vi "Day 1.vi"() -> ()   [LabVIEW 2023]
panel:
  out "top 3":i32
  out "MAX":i32
  in  "Input":string="22243\n11899\n\n1696\n2595\n5331\n6092\n5274\n5641\n1345\n6626\n2005\n6260\n6410\n2092\n3501\n\n3982\n4505\n5836\n6059\n6513\n1151\n\n7002\n6597\n7174\n3618\n4734\n5107\n1388\n6493\n6541\n6440\n5291\n4492\n\n1341\n6520\n8531\n3483\n9221\n2847\n3930\n4012\n\n4074\n2101\n2200\n1333\n2991\n3186\n6711\n2248\n6655\n\n5102\n2672\n2842\n2274\n6828\n3765\n5290\n6004\n7237\n1509\n3128\n1593\n\n8404\n7548\n4075\n8246\n5590\n2107\n1204\n6374\n1865\n5657\n\n62852\n\n10643\n5981\n9631\n1574\n2962\n1021\n9811\n1566\n\n2027\n1193\n1487\n4493\n6215\n3315\n1353\n3703\n3987\n8158\n\n5969\n3824\n4696\n6948\n5098\n1364\n5943\n2489\n3523\n2585\n3242\n5724\n\n2113\n1381\n4067\n2344\n4778\n2645\n3968\n6599\n6451\n4462\n3882\n2312\n3843\n\n294..."
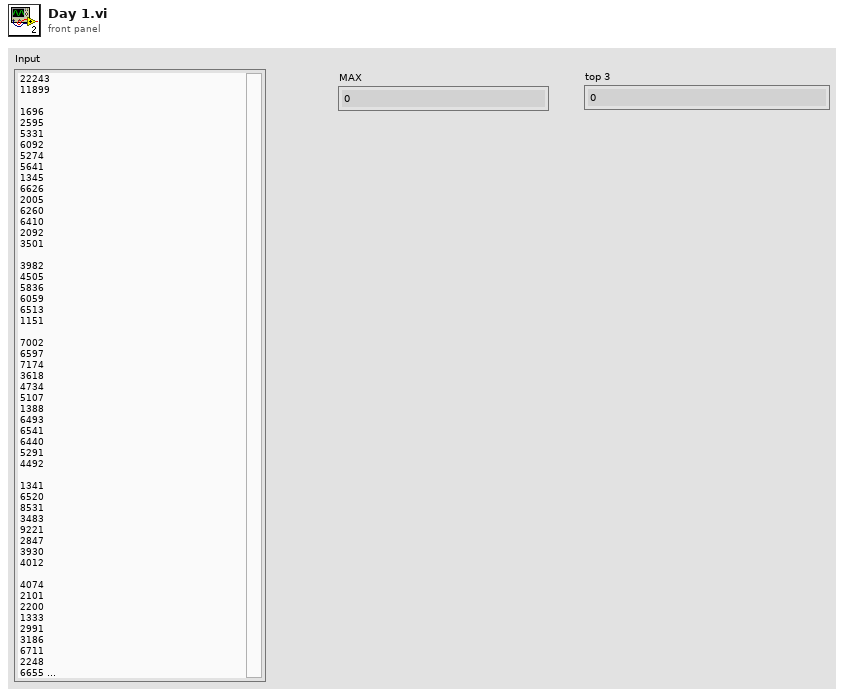
[diagram p1: front panel]
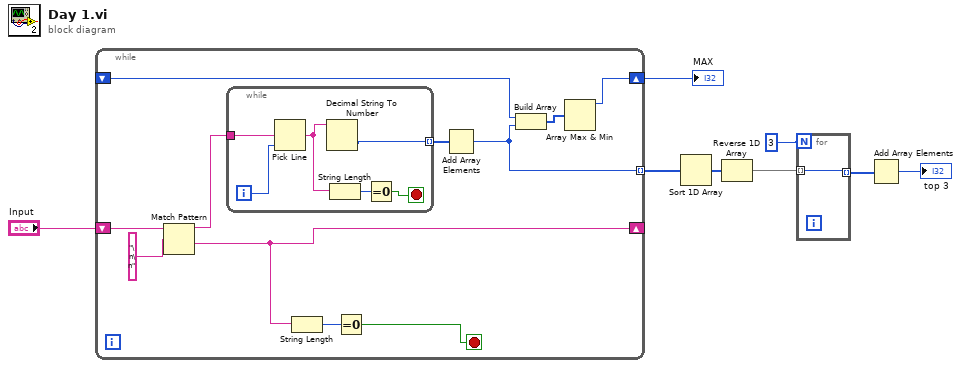
[diagram p0: block diagram]
diagram:
  n1 = while {
    shift-right: [w16] -> _
    shift-left: "Input" -> [w19]
    shift-right: [w11] -> w7
    shift-left: _ -> [w10]
    tunnel: [w9] -> w6 mode=indexing
    stop <- w15 stop-if-true
    n2 = Match Pattern(string=w19, regular expression="\n\n") -> (before substring=w14:string, after substring=w16:string)  [unwired: 1 in, 2 out]
    n3 = while {
      tunnel: w14 -> [w23]
      tunnel: [w24] -> w13 mode=indexing
      i -> [w25]
      stop <- w21 stop-if-true
      n4 = Pick Line(multi-line string=w23, line index=w25) -> (output string=w20:string)  [unwired: 1 in]
      n5 = Decimal String To Number(string=w20) -> (number=w24:i32)  [unwired: 2 in, 1 out]
      n6 = String Length(string=w20) -> (length=w22:i32)
      n7 = Equal To 0?(x=w22) -> (x = 0?=w21:bool)
    }
    n8 = String Length(string=w16) -> (length=w17:i32)
    n9 = Equal To 0?(x=w17) -> (x = 0?=w15:bool)
    n10 = Add Array Elements(numeric array=w13) -> (sum=w9:i32)
    n11 = Build Array(w10, w9) -> (w12:i32[])
    n12 = Array Max & Min(array=w12) -> (max value=w11:i32)  [unwired: 3 out]
  }
  "MAX" <- w7
  n13 = Sort 1D Array(array=w6) -> (sorted array=w5:i32[])
  n14 = Reverse 1D Array(array=w5) -> (reversed array=w4:i32[])
  n15 = for {
    N: 3 -> [_]
    tunnel: w4 -> [w26] mode=indexing
    tunnel: [w26] -> w2 mode=indexing
  }
  n16 = Add Array Elements(numeric array=w2) -> (sum=→"top 3":i32)
